vi "NI VeriStand - Get Target Type.vi"(8 "error in (no error)":errorcluster, 11 "Node U64 ID":T2 format="%.0x") -> (0 "error out":errorcluster, 3 "Operating System":T1)   [LabVIEW 2020, in "Custom Device Offline API.lvlib"]
uses:
  <vilib>/NI VeriStand/Custom Device Offline API/Custom Device Offline API.lvlib
  <vilib>/NI VeriStand/Custom Device API/Custom Device Item Ref.ctl
  <vilib>/NI VeriStand/Custom Device API/Custom Device Target Type.ctl
  NationalInstruments.VeriStand.SystemDefinitionAPI
  NationalInstruments.VeriStand.SystemStorage
  <vilib>/NI VeriStand/Custom Device API/Custom Device API.lvlib
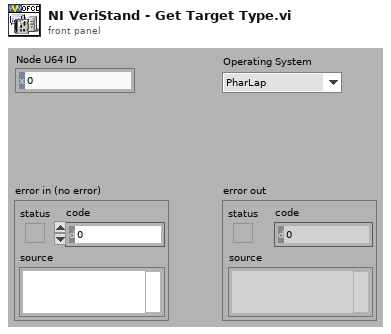
[diagram p1: front panel]
types:
  T1 = typedef "Custom Device API.lvlib/Custom Device Target Type.ctl" = enum16{"PharLap", "VxWorks", "Windows", "Linux_32_ARM", "Linux_x64"}
  T2 = typedef "Custom Device API.lvlib/Custom Device Item Ref.ctl" = u64
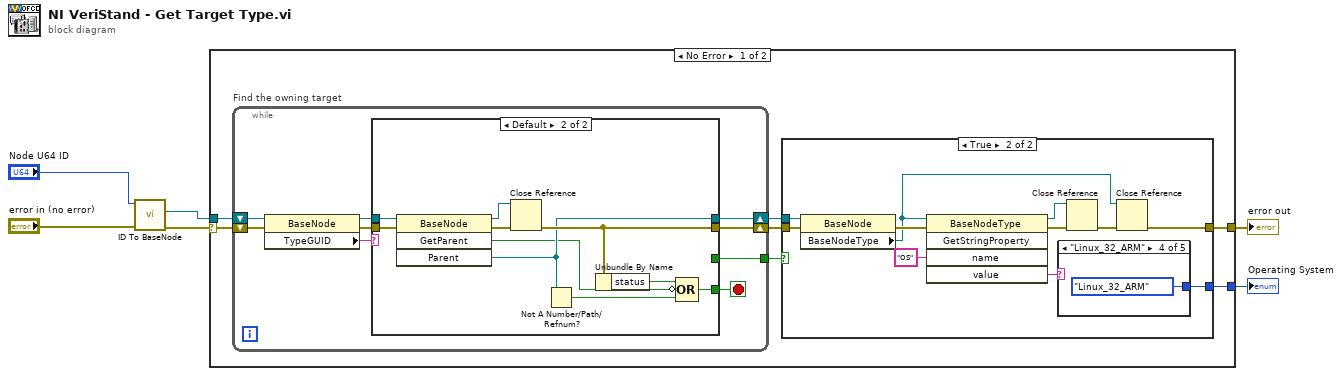
[diagram p0: block diagram]
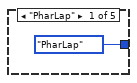
[diagram p3: hidden frame]
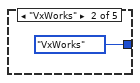
[diagram p4: hidden frame]
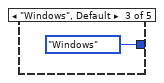
[diagram p5: hidden frame]
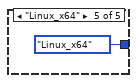
[diagram p6: hidden frame]
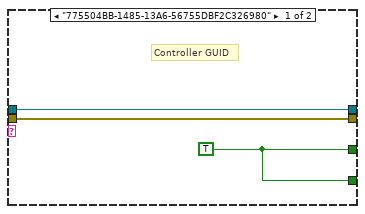
[diagram p7: hidden frame]
diagram:
  n1 = call <vilib>:"ID To BaseNode.vi"("error in (no error)"="error in (no error)", "ID in"="Node U64 ID") -> ("error out"=w4:errorcluster, "BaseNode"=w3:refnum<k24>)  [unwired: 7 in, 1 out]
  n2 = case shown="No Error" w4 {
    selector: w4 -> [w13 w53]
    tunnel: w3 -> [w12 _]
    tunnel: [w7 w53] -> w2
    tunnel: [w8 _] -> w1
    frame No Error {
      n3 = while "Find the owning target" {
        shift-right: [w38] -> w11
        shift-left: w13 -> [w35]
        shift-right: [w37] -> w9
        shift-left: w12 -> [w34]
        tunnel: [w36] -> w10
        stop <- w39 stop-if-true
        n4 = property class="BaseNode"(reference=w34, error in=w35) -> (reference out=w31:refnum<k24>, error out=w32:errorcluster, "TypeGUID"=w33:string)
        n5 = case shown="Default" w33 {
          tunnel: w32 -> [w41 w49]
          tunnel: w31 -> [w42 w48]
          tunnel: [w40 w50] -> w39
          tunnel: [w41 w52] -> w38
          tunnel: [w42 w47] -> w37
          tunnel: [w40 _] -> w36
          frame "775504BB-1485-13A6-56755DBF2C326980" {
            w40 = TRUE
            # "Controller GUID"
          }
          frame Default {
            n6 = invoke class="BaseNode" method="GetParent"(reference=w48, error in=w49) -> (reference out=w45:refnum<k24>, error out=w46:errorcluster, "GetParent"=w43:bool, "Parent"=w47:refnum<k24>)  [unwired: 2 in]
            n7 = Close Reference(reference=w45, error in (no error)=w46) -> (error out=w52:errorcluster)
            n8 = Not A Number/Path/Refnum?(number/path/refnum=w47) -> (NaN/Path/Refnum?=w44:bool)
            n9 = Unbundle By Name(w52) -> ("status"=w51:bool)
            n10 = Compound Arithmetic op=OR(w51, invert w43, w44) -> (w50:bool)
          }
        }
      }
      n11 = case shown="True" w10 {
        tunnel: w11 -> [w14 w25]
        tunnel: w9 -> [_ w23]
        tunnel: [_ w20] -> w8
        tunnel: [w14 w15] -> w7
        frame False {
        }
        frame True {
          n12 = property class="BaseNode"(reference=w23, error in=w25) -> (error out=w24:errorcluster, "BaseNodeType"=w16:refnum<k24>)  [unwired: 1 out]
          n13 = invoke class="BaseNodeType" method="GetStringProperty"(reference=w16, error in=w24, "name"="OS") -> (reference out=w18:refnum<k24>, error out=w19:errorcluster, "value"=w21:string)  [unwired: 2 in, 2 out]
          n14 = case shown="\"Linux_32_ARM\"" w21 {
            tunnel: [Custom_Device_Target_Type."PharLap" ("Operating System") Custom_Device_Target_Type."VxWorks" ("Operating System") Custom_Device_Target_Type."Windows" ("Operating System") Custom_Device_Target_Type."Linux_32_ARM" ("Operating System") Custom_Device_Target_Type."Linux_x64" ("Operating System")] -> w20
            frame "PharLap" {
            }
            frame "VxWorks" {
            }
            frame "Windows", Default {
            }
            frame "Linux_32_ARM" {
            }
            frame "Linux_x64" {
            }
          }
          n15 = Close Reference(reference=w18, error in (no error)=w19) -> (error out=w17:errorcluster)
          n16 = Close Reference(reference=w16, error in (no error)=w17) -> (error out=w15:errorcluster)
        }
      }
    }
    frame Error {
    }
  }
  "error out" <- w2
  "Operating System" <- w1
